vi "Query Counting Mode.vi"(8 "error in (no error)":errorcluster, 11 "VISA resource name":refnum<visa-resource-name>) -> (0 "error out":errorcluster, 2 "output":T1, 3 "VISA resource name out":refnum<visa-resource-name>)   [LabVIEW 2015, in "SR400.lvlib"]
doc: "If j is included, the CM command sets the\ncounting mode. If j is absent, the counting mode is\nreturned.\nj Counting Mode\n0 A,B FOR T PRESET\n1 A-B FOR T PRESET\n2 A+B FOR T PRESET\n3 A FOR B PRESET\nSetting the counter mode also performs a counter\nreset."
uses:
  SR400.lvlib
  Typedefs/Counter Mode.ctl
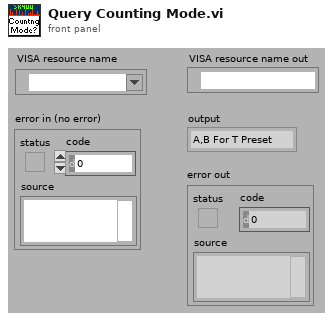
[diagram p1: front panel]
types:
  T1 = typedef "SR400.lvlib/Counter Mode.ctl" = enum16{"A,B For T Preset", "A-B For T Preset", "A+B For T Preset", "A For B Preset"}
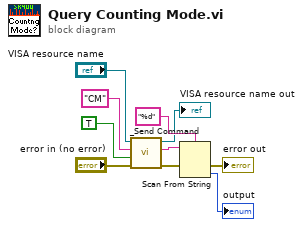
[diagram p0: block diagram]
diagram:
  n1 = call "_Send Command.vi"("error in (no error)"="error in (no error)", "Query? (F)"=TRUE, "Command"="CM" ("command"), "VISA resource name"="VISA resource name") -> ("error out"=w2:errorcluster, "Response"=w3:string, "VISA resource name out"=→"VISA resource name out":refnum<visa-resource-name>)  [unwired: 5 out]
  n2 = Scan From String(format string="%d", input string=w3, error in=w2) -> (error out=→"error out":errorcluster, output 1=→"output":T1)  [unwired: 1 in, 3 out]
